vi "Close stdin.vi"(8 "error in":errorcluster, 11 "connection in":refnum<class "Low Level Connection.lvclass">) -> (0 "error out":errorcluster, 3 "connection out":refnum<class "Low Level Connection.lvclass">)   [LabVIEW 2020, in "NI_SFTP.lvlib" / "Low Level Connection.lvclass"]
uses:
  <vilib>/net/SFTP/Low Level Connection/Low Level Connection.lvclass
  <vilib>/net/SFTP/Low Level Connection/Low Level Connection.lvclass/Low Level Connection.ctl
  <vilib>/Subprocess/Buffered Subprocess/Buffered Subprocess.lvclass
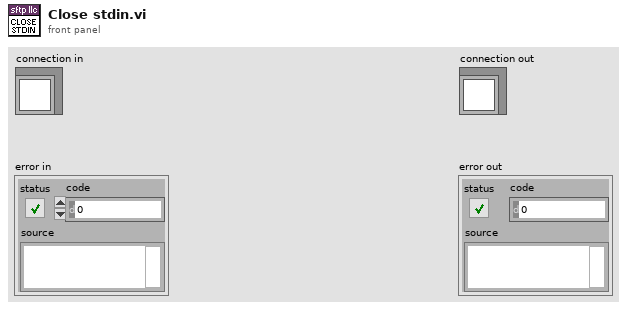
[diagram p1: front panel]
types:
  T1 = cluster{"subprocess":refnum<class "Buffered Subprocess.lvclass">, "read stdout":refnum<class "Bytestream.lvclass">}
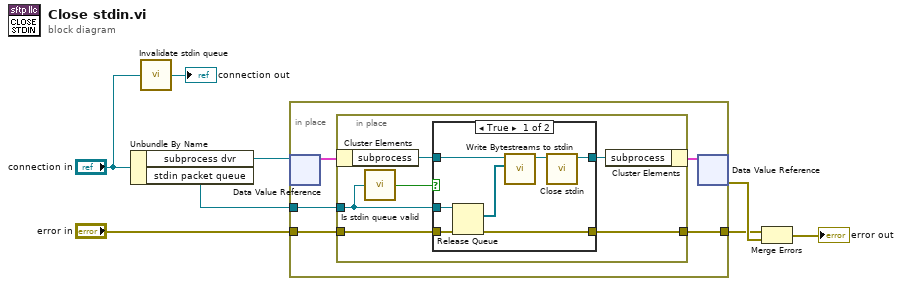
[diagram p0: block diagram]
diagram:
  n1 = Unbundle By Name("connection in") -> ("subprocess dvr"=w4:refnum<data-value>, "stdin packet queue"=w3:refnum<queue>)
  n2 = call <vilib>:"Invalidate stdin queue.vi"("connection in"="connection in") -> ("connection out"=→"connection out":refnum<class "Low Level Connection.lvclass">)
  n3 = in-place {
    in-place-border: "error in" -> [w11]
    in-place-border: [w13] -> w1
    in-place-border: w3 -> [w12]
    n4 = in-place-dvr #1(w4) -> (w10:T1)  [unwired: 1 out]
    n5 = in-place {
      in-place-border: [w16] -> w13
      in-place-border: w12 -> [w15]
      in-place-border: w11 -> [w19]
      n6 = in-place-cluster #2(w10) -> ("subprocess"=w18:refnum<class "Buffered Subprocess.lvclass">)
      n7 = call <vilib>:"Is stdin queue valid.vi"("stdin packet queue"=w15) -> ("valid?"=w14:bool)
      n8 = case shown="True" w14 {
        tunnel: w15 -> [w23 _]
        tunnel: w19 -> [w22 w27]
        tunnel: w18 -> [w24 w28]
        tunnel: [w21 w28] -> w17
        tunnel: [w20 w27] -> w16
        frame True {
          n9 = Release Queue(queue=w23, error in (no error)=w22) -> (remaining elements=w26:refnum<class "Bytestream.lvclass">[], error out=w20:errorcluster)  [unwired: 1 in, 1 out]
          n10 = call <vilib>:"Write Bytestreams to stdin.vi"("data"=w26, "subprocess in"=w24) -> ("subprocess out"=w25:refnum<class "Buffered Subprocess.lvclass">)  [unwired: 9 in]
          n11 = call <vilib>:"Close stdin.vi"("subprocess in"=w25) -> ("subprocess out"=w21:refnum<class "Buffered Subprocess.lvclass">)  [unwired: 10 in]
        }
        frame False {
        }
      }
      n12 = in-place-cluster #2("subprocess"=w17) -> (w9:T1)
    }
    n13 = in-place-dvr #1(w9) -> (w2:errorcluster)  [unwired: 1 out]
  }
  n14 = Merge Errors(w1, w2) -> (→"error out":errorcluster)
